vi "Data Conversion - Prepare Waveforms for Upload (2D I16 to LEndian U8).vi"(10 "Multichannel Waveform (Signed 16 Bit - 2D Array)":i16[][](array[numeric])) -> (2 "Unsigned Byte Array":u8[](array[numeric]))   [LabVIEW 2017, in "Communications Library.lvlib"]
doc: "Converts a 2D array of 16 bit integers into an array of bytes in little-endian format."
uses:
  Communications Library.lvlib
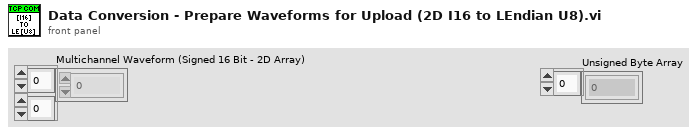
[diagram p1: front panel]
types:
  T1 = enum16{"Little-Endian (LSBF)", "Big-Endian (MSBF)"}
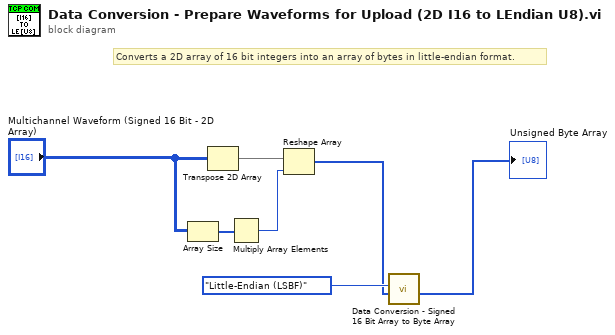
[diagram p0: block diagram]
diagram:
  # "Converts a 2D array of 16 bit integers into an array of bytes in little-endian format."
  n1 = Array Size(array="Multichannel Waveform (Signed 16 Bit - 2D Array)") -> (size(s)=w7:i32[])
  n2 = Transpose 2D Array(2D array="Multichannel Waveform (Signed 16 Bit - 2D Array)") -> (transposed array=w2:i16[][])
  n3 = Multiply Array Elements(1:w7) -> (0:w6:i32)
  n4 = Reshape Array(w2, w6) -> (w1:i16[])
  n5 = call "Data Conversion - Signed 16 Bit Array to Byte Array.vi"("16 Bit Array (Signed) In"=w1, "Byte Order"=T1."Little-Endian (LSBF)") -> ("Byte Array (Unsigned) Out"=→"Unsigned Byte Array":u8[])  [unwired: 9 in]
